vi "Activate AllHW.vi"(8 "error in (no error)":errorcluster, 11 "BME_DG_System in":refnum<class "BME_DG_System.lvclass">) -> (0 "error out":errorcluster, 3 "BME_DG_System out":refnum<class "BME_DG_System.lvclass">)   [LabVIEW 2009, in "POLARIS BME DG.lvlib" / "BME_DG_System.lvclass"]
doc: "Activates all DGs, first the slaves and when the master\n\nATTENTION: If You have reseted output modulo counter, ALL channels fires a common shot after activation of master. If our plant needs some cool down breaks, make sure to implement they.\n\n\n\n---------------\n\nauthor: Alexander Kessler, Helmholtz-Institut-Jena \nmaintainer: Alexander Kessler: alexander.kessler@uni-jena.de\n\n\nLicense Agreement for this software:\n\nCopyright (C)\nHelmholtz-Institut-Jena\nFröbelsteg 3\n07743 Jena\nGermany\n\nContact: alexander.kessler@uni-jena.de\n\nThis program is free software; you can redistribute it and/or modify it under the terms of the GNU General Public License as published by the Free Software Foundation; either version 2 of the license, or (at your option) any later version.\n\nThis program is distributed in the hope that it will be useful, but WITHOUT ANY WARRANTY; without even the implied warranty of MERCHANTABILITY or FITNESS FOR A PARTICULAR PURPOSE. See the GNU General License for more details (http://www.gnu.org)."
uses:
  BME_DG_System.lvclass
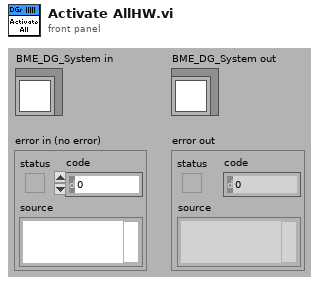
[diagram p1: front panel]
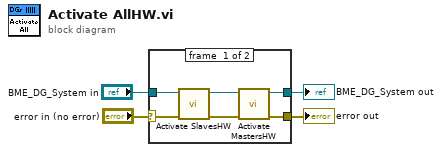
[diagram p0: block diagram]
diagram:
  n1 = case shown="No Error" "error in (no error)" {
    selector: "error in (no error)" -> [w10 w12]
    tunnel: [w8 w12] -> w3
    tunnel: [w5 w11] -> w1
    tunnel: "BME_DG_System in" -> [w7 w11]
    frame #0 {
      n2 = call "Activate SlavesHW.vi"("error in (no error)"=w10, "BME_DG_System in"=w7) -> ("error out"=w9:errorcluster, "BME_DG_System out"=w6:refnum<class "BME_DG_System.lvclass">)  [unwired: 8 in]
      n3 = call "Activate MastersHW.vi"("error in (no error)"=w9, "BME_DG_System in"=w6) -> ("error out"=w8:errorcluster, "BME_DG_System out"=w5:refnum<class "BME_DG_System.lvclass">)  [unwired: 8 in]
    }
    frame #1 {
    }
  }
  "error out" <- w3
  "BME_DG_System out" <- w1
